vi "Test Image Acquisition.vi"() -> ()   [LabVIEW 2017]
uses:
  BonTechWrapperLibrary.dll
  <vilib>/vision/Image Controls.llb/IMAQ Image.ctl
panel:
  out "error out":errorcluster
  out "Image":T1(plugin-control)
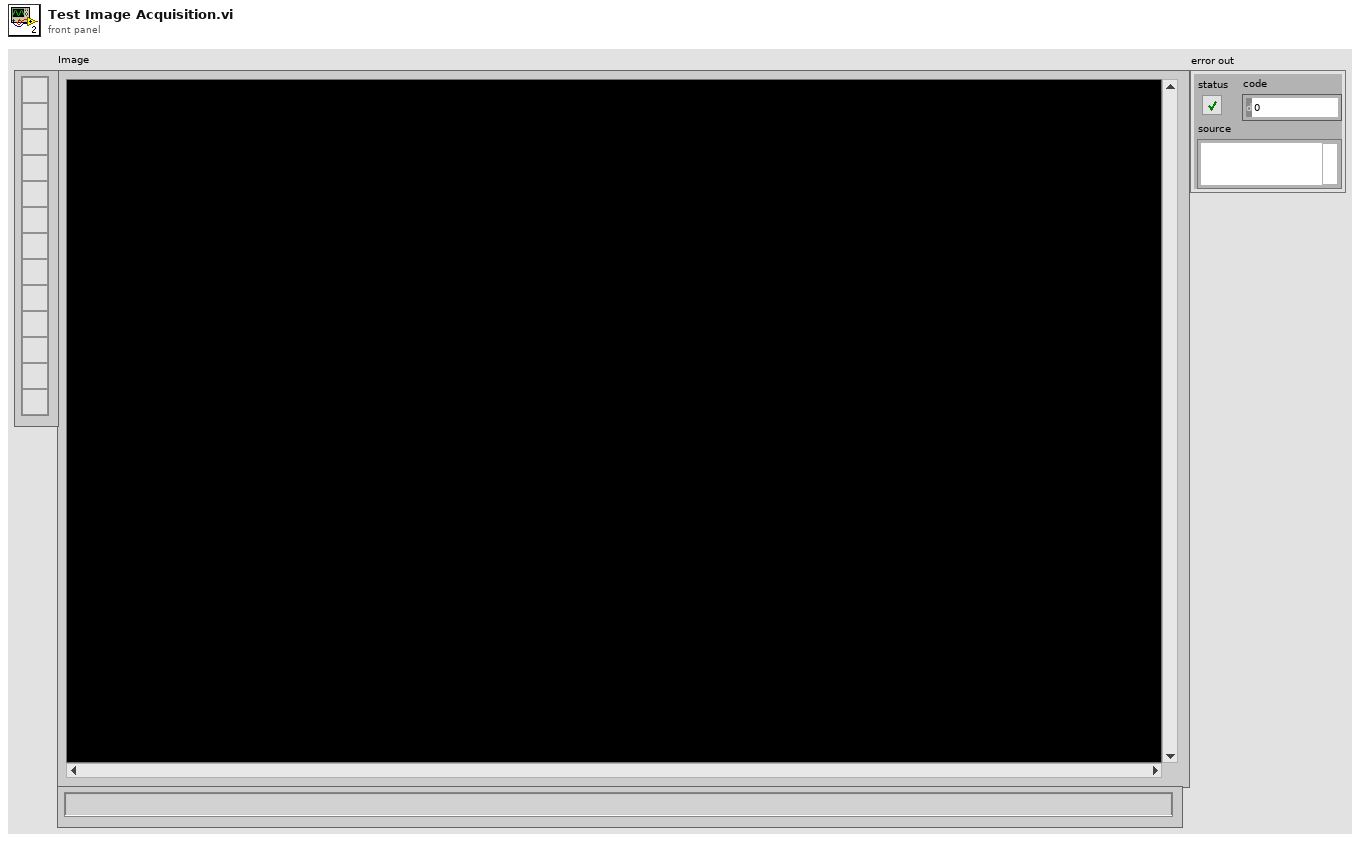
[diagram p1: front panel]
types:
  T1 = typedef "IMAQ Image.ctl" = refnum<image>
  T2 = typedef "Image Type" = u32
  T3 = enum32{"Map Pixel Pointer", "Unmap Pixel Pointer", "Get Pixels Infos"}
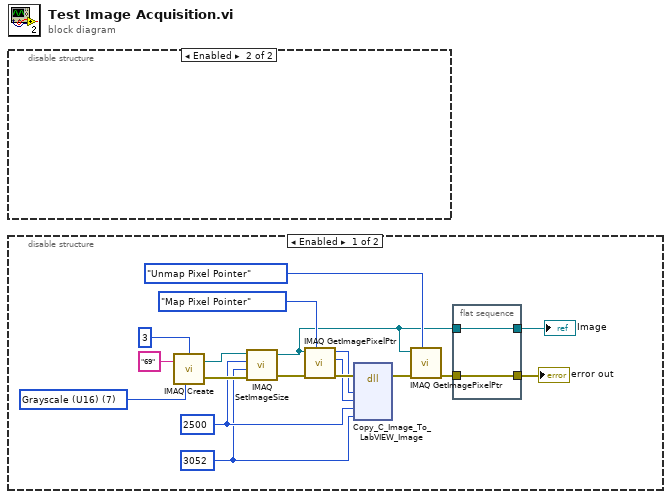
[diagram p0: block diagram]
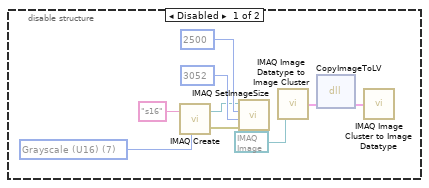
[diagram p3: hidden frame]
diagram:
  n1 = disable-structure shown="Enabled" {
    frame Disabled {
      w3 = T2 7 items=["Grayscale (U8)", "Grayscale (I16)", "Grayscale (SGL)", "Complex (CSG)", "RGB (U32)", "HSL (U32)", "RGB (U64)", "Grayscale (U16)"] ("Image Type")
      n2 = call "IMAQ Create"("Image Name"="s16", "Image Type"=w3) -> ("New Image"=w2:T1, "error out"=w9:errorcluster)  [unwired: 3 in]
      n3 = call "IMAQ SetImageSize"("error in (no error)"=w9, "Y Resolution"=3052, "X Resolution"=2500, "Image"=w2) -> ()  [unwired: 1 in, 2 out]
      n4 = call "IMAQ Image Datatype to Image Cluster.vi"("Image"=T1 refnum) -> ("Image (dup)"=w6:cluster{string, u32})
      n5 = dll-call lib="E:/GitHub/BonTechWrapperLibrary/BonTechWrapperLibrary/x64/Release/BonTechWrapperLibrary.dll" fn="CopyImageToLV"("arg1"=w6) -> ("arg1"=w5:cluster{string, u32})  [unwired: 4 in, 2 out]
      n6 = call "IMAQ Image Cluster to Image Datatype.vi"("Image"=w5) -> ()  [unwired: 1 out]
    }
    frame Enabled {
    }
  }
  n7 = disable-structure shown="Enabled" {
    frame Enabled {
      w20 = T2 7 items=["Grayscale (U8)", "Grayscale (I16)", "Grayscale (SGL)", "Complex (CSG)", "RGB (U32)", "HSL (U32)", "RGB (U64)", "Grayscale (U16)"] ("Image Type")
      w16 = 3052 ("Y Resolution")
      w17 = 2500 ("X Resolution")
      n8 = call "IMAQ Create"("Border Size"=3, "Image Name"="69", "Image Type"=w20) -> ("New Image"=w21:T1, "error out"=w18:errorcluster)  [unwired: 2 in]
      n9 = call "IMAQ SetImageSize"("error in (no error)"=w18, "Y Resolution"=w16, "X Resolution"=w17, "Image"=w21) -> ("error out"=w15:errorcluster, "Image Out"=w13:T1)  [unwired: 1 in]
      n10 = call "IMAQ GetImagePixelPtr"("Function"=T3."Map Pixel Pointer", "error in (no error)"=w15, "Image"=w13) -> ("error out"=w25:errorcluster, "LineWidth(Pixels)"=w22:i32, "Pixel Pointer out"=w23:u64)  [unwired: 3 in, 3 out]
      n11 = dll-call lib="E:/GitHub/BonTechWrapperLibrary/BonTechWrapperLibrary/x64/Release/BonTechWrapperLibrary.dll" fn="Copy_C_Image_To_LabVIEW_Image"(error in=w25, "LVImgPtr"=w23, "LVLineWidth"=w22, "LVWidth"=w17, "LVHeight"=w16) -> (error out=w24:errorcluster)  [unwired: 7 in, 1 out]
      n12 = call "IMAQ GetImagePixelPtr"("Function"=T3."Unmap Pixel Pointer", "error in (no error)"=w24, "Image"=w13) -> ("error out"=w14:errorcluster)  [unwired: 3 in, 5 out]
      n13 = flat-sequence {
        tunnel: w14 -> [w29]
        tunnel: [w29] -> w12
        tunnel: w13 -> [w28]
        tunnel: [w28] -> w10
        frame #0 {
        }
      }
      "error out" <- w12
      "Image" <- w10
    }
    frame Disabled {
    }
  }
